vi "trace_counts_to_volts.vi"(10 "Counts In":i16[](array[numeric]), 11 "Voltage Range":dbl) -> (3 "Voltage Out":dbl[](array[numeric]))   [LabVIEW 2013]
panel:
  out "Waveform Graph":i16[](graph)
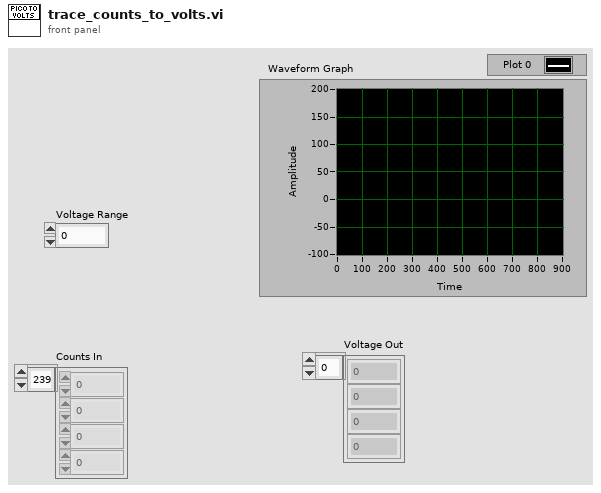
[diagram p1: front panel]
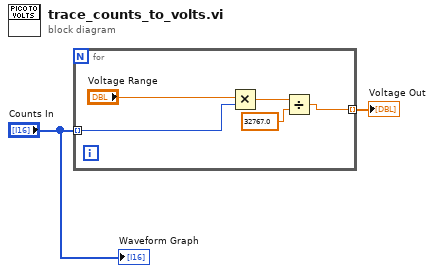
[diagram p0: block diagram]
diagram:
  n1 = for {
    tunnel: "Counts In" -> [w5] mode=indexing
    tunnel: [w4] -> w2 mode=indexing
    n2 = Multiply(x="Voltage Range", y=w5) -> (x*y=w7:dbl)
    n3 = Divide(x=w7, y=32767.0) -> (x/y=w4:dbl)
  }
  "Voltage Out" <- w2
  "Waveform Graph" <- "Counts In"
